vi "Read product config.vi"(8 "error in (no error)":errorcluster) -> (0 "error out":errorcluster, 3 "Item Names out":string[][](array[string]))   [LabVIEW 2020, in "Productos.lvlib"]
uses:
  Productos.lvlib
  <vilib>/Utility/xml.llb/Read From XML File(string).vi
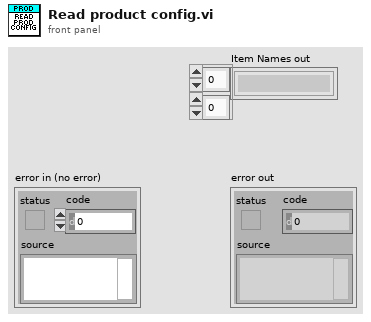
[diagram p1: front panel]
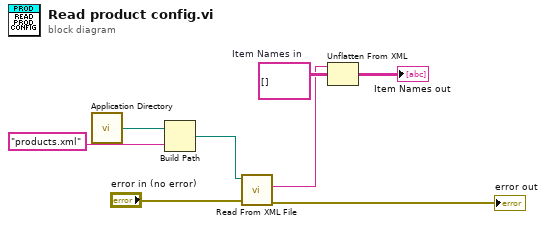
[diagram p0: block diagram]
diagram:
  w4 = string[][] []  # Item Names in
  n1 = call <vilib>:"Application Directory.vi"() -> ("Application Directory"=w8:path)
  n2 = Build Path(base path=w8, name or relative path="products.xml") -> (appended path=w2:path)
  n3 = call-poly <vilib>:"Read From XML File.vi"("error in (no error)"="error in (no error)", "XML File Path"=w2) -> ("error out"=→"error out":errorcluster, "XML Elements"=w1:string)  [unwired: 7 in, 1 out]
  n4 = Unflatten From XML(xml string=w1, type=w4) -> (value=→"Item Names out":string[][])  [unwired: 1 in, 1 out]
